vi "ini_sesion.vi"(8 "error in (no error)":errorcluster, 10 "trig out port":string="PXI_Trig0", 11 "5785_2_x_1600MHz in":refnum<class "5785_2_x_1600MHz.lvclass">) -> (0 "error out":errorcluster, 3 "5785_2_x_1600MHz out":refnum<class "5785_2_x_1600MHz.lvclass">)   [LabVIEW 2021, in "5785_2_x_1600MHz.lvclass"]
uses:
  5785_2_x_1600MHz.lvclass
  5785_2_x_1600MHz.lvclass/5785_2_x_1600MHz.ctl
  <instrlib>/FlexRIO/API/Host/v1/NI FlexRIO/API/Reference Clock Source.ctl
  <vilib>/FPGAPlugInAG/PXIe-5785 (KU060)/niLvFpga_Open_PXIe-5785 (KU060).vi
  <vilib>/rvi/interface/common/dynamic/niFpgaDynamicAddResources.vi
  <instrlib>/FlexRIO/API/Host/v1/NI FlexRIO/API/Configure Reference Clock.vi
  <vilib>/Utility/error.llb/Error Cluster From Error Code.vi
  <vilib>/rvi/errors/niLvFpgaAdjustHostInterfaceError.vi
  <vilib>/rvi/interface/common/niFpgaWaitOnOcc.vi
  <instrlib>/FlexRIO/API/Host/v1/NI FlexRIO/API/Get Property Reference - Fpga Small.vi
  <vilib>/rvi/interface/nirviOpenFPGA/nirviOpenFPGA.xnode
  FPGA Bitfiles/5785_multi emitter_2_x_1_6G.lvbitx
  FPGA Bitfiles/5785_IQ_gen_2_x_1.6GHz_max_mod_8_and_4.lvbitx
  <vilib>/rvi/interface/nirviReadWriteControl/nirviReadWriteControl.xnode
  <vilib>/rvi/interface/nirviMethod/nirviMethod.xnode
  <instrlib>/FlexRIO/API/Host/v1/NI FlexRIO API v1.lvlib
  <resource>/objmgr/niflexrioapiStream.rc
  <resource>/objmgr/niflexrioapi.rc
  <vilib>/FPGAPlugInAG/Dynamic/niLvFpga_ConfigureFifo_Dynamic.vi
  <vilib>/rvi/errors/niLvFpgaMergeErrorWithErrorCode.vi
  <resource>/objmgr/niflexrioapiChannel.rc
  <vilib>/FPGAPlugInAG/Dynamic/niLvFpga_StopFifo_Dynamic.vi
  NiFpgaLv.dll
  <vilib>/rvi/interface/Simulation/niFpgaSimulationCallBeginRW.vi
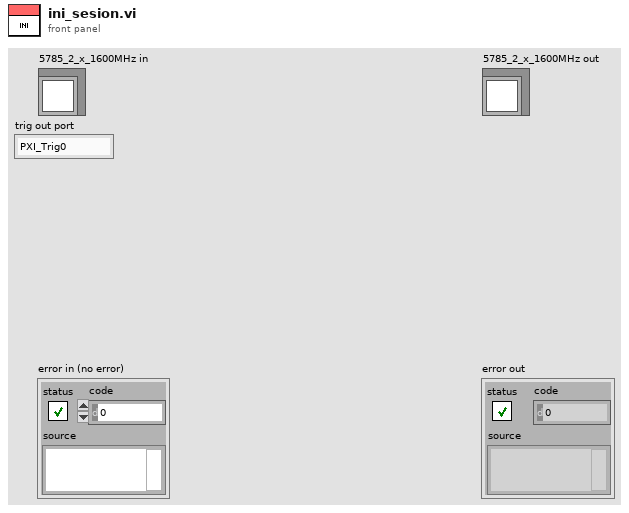
[diagram p1: front panel]
types:
  T1 = typedef "nirio_resource_hc.ctl" = tag
  T2 = typedef "NI FlexRIO API v1.lvlib/Reference Clock Source.ctl" = i32
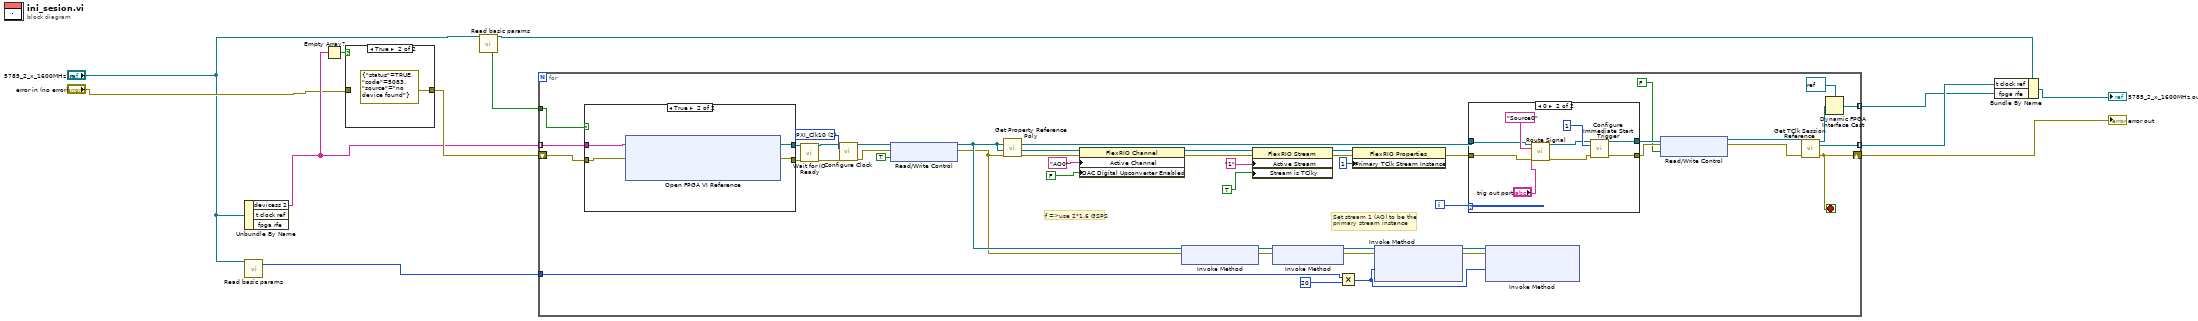
[diagram p0: block diagram]
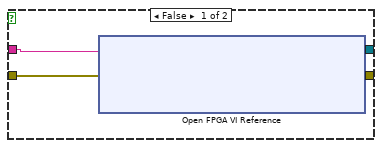
[diagram p3: hidden frame]
diagram:
  n1 = Unbundle By Name("5785_2_x_1600MHz in") -> ("devicess 2"=w8:T1[])  [unwired: 2 out]
  n2 = call-dynamic "Read basic params.vi"("device_type in"="5785_2_x_1600MHz in") -> ("buffer size"=w9:u32)  [unwired: 11 in, 7 out]
  n3 = Empty Array?(array=w8) -> (empty?=w11:bool)
  n4 = case shown="True" w11 {
    tunnel: [w13 errorcluster {"status"=TRUE, "code"=5083, "source"="no device found"} ("error in (no error)")] -> w10
    tunnel: "error in (no error)" -> [w13 _]
    frame False {
    }
    frame True {
    }
  }
  n5 = call-dynamic "Read basic params.vi"("device_type in"="5785_2_x_1600MHz in") -> ("use arb files"=w1:bool, "device_type out"=w2:refnum<class "5785_2_x_1600MHz.lvclass">)  [unwired: 11 in, 6 out]
  n6 = for {
    shift-right: [w34] -> w6
    shift-left: w10 -> [w49]
    tunnel: [w54] -> w12 mode=indexing
    tunnel: w8 -> [w38] mode=indexing
    tunnel: w9 -> [w26]
    tunnel: [w24] -> w4 mode=indexing
    tunnel: w1 -> [w22]
    i -> [w52]
    stop <- w34 stop-if-true
    w37 = T2 2 items=["Default", "Onboard", "PXI_Clk10", "External", "None", "Baseboard Reference"] ("reference clock source")
    # "f =>use 2*1.6 GSPS"
    # "Set stream 1 (AO) to be the\nprimary stream instance"
    n7 = case shown="True" w22 {
      tunnel: [w63 w65] -> w51
      tunnel: [w62 w64] -> w50
      tunnel: w49 -> [w61 w66]
      tunnel: w38 -> [w60 w67]
      frame False {
        n8 = xnode "Open FPGA VI Reference"("error in"=w61, "resource name"=w60) -> ("FPGA VI Reference Out"=w63:refnum<k20>, "error out"=w62:errorcluster)
      }
      frame True {
        n9 = xnode "Open FPGA VI Reference"("error in"=w66, "resource name"=w67) -> ("FPGA VI Reference Out"=w65:refnum<k20>, "error out"=w64:errorcluster)
      }
    }
    n10 = call <instrlib>:"Wait for IO Ready.vi"("fpga interface in"=w51, "error in"=w50) -> ("fpga interface out"=w36:refnum<k20>, "error out"=w35:errorcluster)  [unwired: 10 in, 2 out]
    n11 = call-poly <instrlib>:"Configure Clock.vi"("fpga interface in"=w36, "reference clock source"=w37, "error in"=w35) -> ("fpga interface out"=w21:refnum<k20>, "error out"=w19:errorcluster)  [unwired: 11 in]
    n12 = xnode "Read/Write Control"("FPGA VI Reference In"=w21, "error in"=w19, "reset system clock"=TRUE) -> ("FPGA VI Reference Out"=w20:refnum<k20>, "error out"=w18:errorcluster)
    n13 = call-poly <instrlib>:"Get Property Reference Poly.vi"("error in (no error)"=w18, "fpga interface in"=w20) -> ("error out"=w41:errorcluster, "property reference"=w42:refnum<k20>)  [unwired: 4 in, 1 out]
    n14 = property class="FlexRIO Channel"(reference=w42, error in=w41, "Active Channel"="AO0", "DAC Digital Upconverter Enabled"=FALSE ("Analog Output:DAC Digital Upconverter Enabled")) -> (reference out=w40:refnum<k20>, error out=w39:errorcluster)
    n15 = xnode "Invoke Method"("FPGA VI Reference In"=w20, "error in"=w18) -> ("FPGA VI Reference Out"=w29:refnum<k20>, "error out"=w30:errorcluster)
    n16 = property class="FlexRIO Stream"(reference=w40, error in=w39, "Active Stream"="1", "Stream is TClky"=TRUE ("Configuration:Stream is TClky")) -> (reference out=w57:refnum<k20>, error out=w56:errorcluster)
    n17 = xnode "Invoke Method"("FPGA VI Reference In"=w29, "error in"=w30) -> ("FPGA VI Reference Out"=w27:refnum<k20>, "error out"=w28:errorcluster)
    n18 = Multiply(x=w26, y=u32 20) -> (x*y=w46:u32)
    n19 = property class="FlexRIO Properties"(reference=w57, error in=w56, "Primary TClk Stream Instance"=1 ("Device:Primary TClk Stream Instance")) -> (error out=w53:errorcluster)  [unwired: 1 out]
    n20 = xnode "Invoke Method"("FPGA VI Reference In"=w27, "error in"=w28, "Requested Depth"=w46) -> ("FPGA VI Reference Out"=w48:refnum<k20>, "error out"=w47:errorcluster)  [unwired: 1 out]
    n21 = case shown="0" w52 {
      tunnel: w20 -> [w69 w74]
      tunnel: [w69 w77] -> w33
      tunnel: [w68 w76] -> w32
      tunnel: w53 -> [w68 w73]
      frame 1, Default {
      }
      frame 0 {
        n22 = call <instrlib>:"Route Signal.vi"("fpga interface in"=w74, "source"="Source0", "destination"="trig out port", "error in"=w73) -> ("fpga interface out"=w72:refnum<k20>, "error out"=w71:errorcluster)  [unwired: 9 in, 1 out]
        n23 = call <instrlib>:"Configure Immediate Start Trigger.vi"("fpga interface in"=w72, "trigger instance"=u32 1, "error in"=w71) -> ("fpga interface out"=w77:refnum<k20>, "error out"=w76:errorcluster)  [unwired: 10 in, 1 out]
      }
    }
    n24 = xnode "Invoke Method"("FPGA VI Reference In"=w48, "error in"=w47, "Requested Depth"=w46) -> ()  [unwired: 3 out]
    n25 = xnode "Read/Write Control"("FPGA VI Reference In"=w33, "error in"=w32, "reset system clock"=FALSE) -> ("FPGA VI Reference Out"=w16:refnum<k20>, "error out"=w15:errorcluster)
    n26 = call <instrlib>:"Get TClk Session Reference.vi"("fpga interface in"=w16, "error in"=w15) -> ("fpga interface out"=w25:refnum<k20>, "tclk session reference"=w54:refnum<k20>, "error out"=w34:errorcluster)  [unwired: 11 in]
    n27 = Dynamic FPGA Interface Cast(Session In=refnum<k20> refnum ("FPGA VI Reference Out"), Type=w25) -> (Session Out=w24:refnum<k20>)
  }
  "error out" <- w6
  n28 = Bundle By Name(cluster=w2, "t clock ref"=w12, "fpga rfe"=w4) -> (→"5785_2_x_1600MHz out":refnum<class "5785_2_x_1600MHz.lvclass">)
